vi "Disconnect Wire from Terminal.vi"(5 "Remove Loose Ends":bool, 7 "Clean Up wire":bool=TRUE, 8 "error in":errorcluster, 11 "Terminal in":refnum<vi>) -> (0 "error out":errorcluster, 1 "Wire valid?":bool, 2 "Wire Out":refnum<vi>, 3 "Terminal out":refnum<vi>, 4 "Wire Terminals[]":refnum<vi>[](array[refnum]))   [LabVIEW 2023]
doc: "Takes a terminal referneces and disconnects wire (if any), and cleans up remaining wire if desired.\n\nWire output terminal may be invalide"
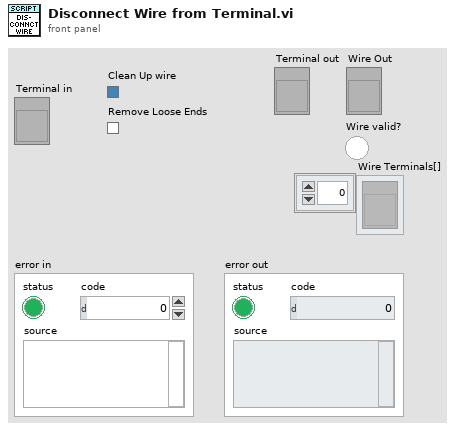
[diagram p1: front panel]
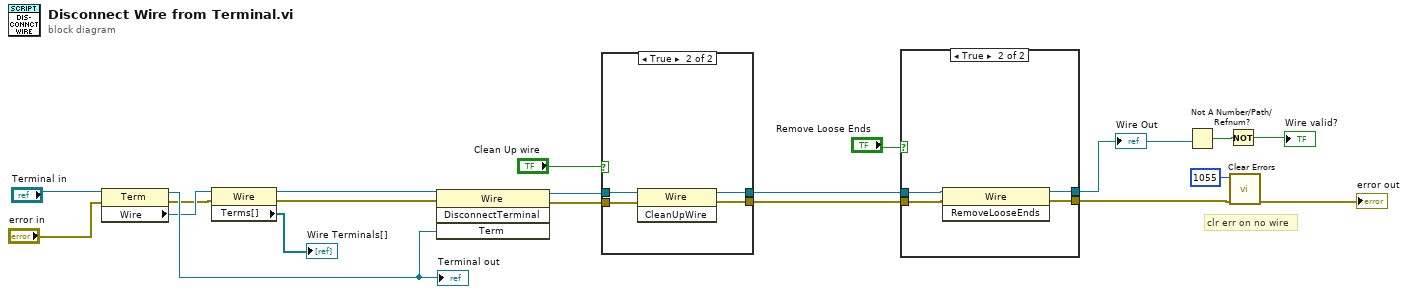
[diagram p0: block diagram]
diagram:
  # "clr err on no wire"
  n1 = property class="Term"(reference="Terminal in", error in="error in") -> (reference out=w17:refnum<vi>, error out=w6:errorcluster, "Wire"=w8:refnum<vi>)
  "Terminal out" <- w17
  n2 = property class="Wire"(reference=w8, error in=w6) -> (reference out=w7:refnum<vi>, error out=w5:errorcluster, "Terms[]"=→"Wire Terminals[]":refnum<vi>[])
  n3 = invoke class="Wire" method="DisconnectTerminal"(reference=w7, error in=w5, "Term"=w17) -> (reference out=w4:refnum<vi>, error out=w3:errorcluster)  [unwired: 1 in, 2 out]
  n4 = case shown="True" "Clean Up wire" {
    tunnel: [w22 w26] -> w11
    tunnel: w3 -> [w22 w25]
    tunnel: w4 -> [w21 w24]
    tunnel: [w21 w23] -> w12
    frame False {
    }
    frame True {
      n5 = invoke class="Wire" method="CleanUpWire"(reference=w24, error in=w25) -> (reference out=w23:refnum<vi>, error out=w26:errorcluster)  [unwired: 1 in, 1 out]
    }
  }
  n6 = case shown="True" "Remove Loose Ends" {
    tunnel: w12 -> [w28 w32]
    tunnel: w11 -> [w27 w31]
    tunnel: [w28 w30] -> w2
    tunnel: [w27 w29] -> w1
    frame False {
    }
    frame True {
      n7 = invoke class="Wire" method="RemoveLooseEnds"(reference=w32, error in=w31) -> (reference out=w30:refnum<vi>, error out=w29:errorcluster)  [unwired: 1 in, 1 out]
    }
  }
  "Wire Out" <- w2
  n8 = Not A Number/Path/Refnum?(number/path/refnum=w2) -> (NaN/Path/Refnum?=w14:bool)
  n9 = Not(x=w14) -> (.not. x?=→"Wire valid?":bool)
  n10 = call <vilib>:"Clear Errors.vi"("error in (no error)"=w1, "specific error code to clear (0: all)"=1055) -> ("error out"=→"error out":errorcluster)  [unwired: 4 in, 1 out]
